vi "setUp.vi"(8 "error in (no error)":errorcluster, 11 "reference in":refnum<class "Test TCP Stream Initiator Connect.lvclass">) -> (0 "error out":errorcluster, 3 "reference out":refnum<class "Test TCP Stream Initiator Connect.lvclass">)   [LabVIEW 2020, in "Test TCP Stream Initiator Connect.lvclass"]
doc: "setUp runs prior to the test method during test execution. Use this method to initialize any object data required by your tests."
uses:
  Test TCP Stream Initiator Connect.lvclass
  <vilib>/addons/_JKI Toolkits/VI Tester/TestCase.llb/TestCase.lvclass
  Source/Protocols/TCP Strategy/TCP Stream Initiator/TCP Stream Initiator.lvclass
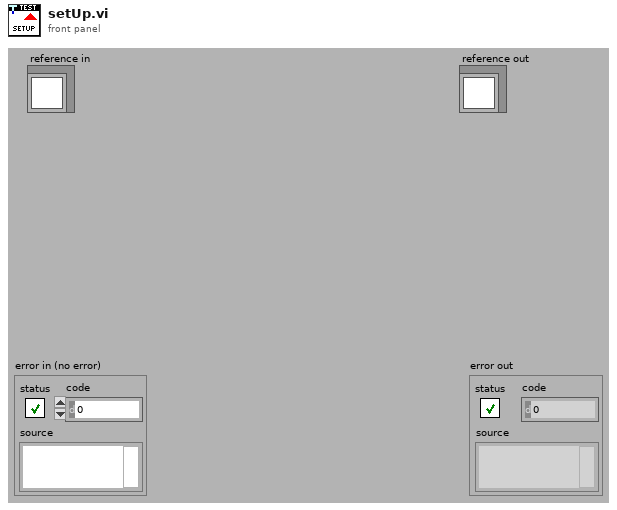
[diagram p1: front panel]
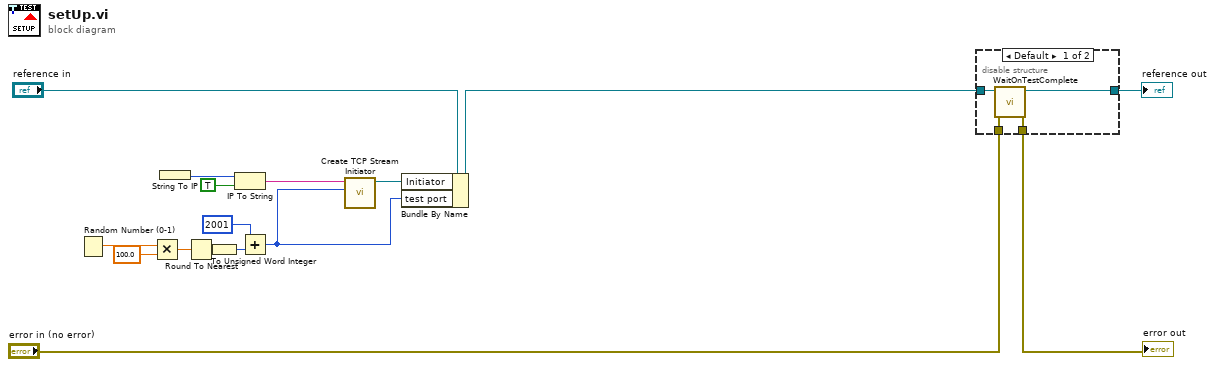
[diagram p0: block diagram]
diagram:
  n1 = Random Number (0-1)() -> (number: 0 to 1=w7:dbl)
  n2 = Multiply(x=w7, y=100.0) -> (x*y=w5:dbl)
  n3 = String To IP() -> (0:w9:u32)  [unwired: 1 in]
  n4 = Round To Nearest(number=w5) -> (nearest integer value=w4:dbl)
  n5 = To Unsigned Word Integer(number=w4) -> (unsigned 16bit integer=w1:u16)
  n6 = IP To String(1:TRUE ("dot notation? (F)"), 2:w9) -> (0:w8:string)
  n7 = Add(x=u16 2001 ("Port"), y=w1) -> (x+y=w2:u16)
  n8 = call "Create TCP Stream Initiator.vi"("Remote Port"=w2, "Remote Address"=w8) -> ("TCP Stream Initiator"=w11:refnum<class "TCP Stream Initiator.lvclass">)  [unwired: 9 in]
  n9 = Bundle By Name(cluster="reference in", "Initiator"=w11, "test port"=w2) -> (w12:refnum<class "Test TCP Stream Initiator Connect.lvclass">)
  n10 = disable-structure shown="Default" {
    disable-tunnel: "error in (no error)" -> [w20 w21]
    disable-tunnel: [w19 w21] -> w15
    disable-tunnel: [w18 w22] -> w13
    disable-tunnel: w12 -> [w17 w22]
    frame condition #0 (active) {
      n11 = call <vilib>:"WaitOnTestComplete.vi"("error in (no error)"=w20, "TestCase in"=w17) -> ("error out"=w19:errorcluster, "TestCase out"=w18:refnum<class "Test TCP Stream Initiator Connect.lvclass">)  [unwired: 8 in]
    }
    frame condition #1 {
    }
  }
  "error out" <- w15
  "reference out" <- w13
